vi "二进制文件读取.vi"() -> ()   [LabVIEW 2018]
panel:
  out "数据 2":i32[](array[numeric])
  in  "path":path caption="路径"
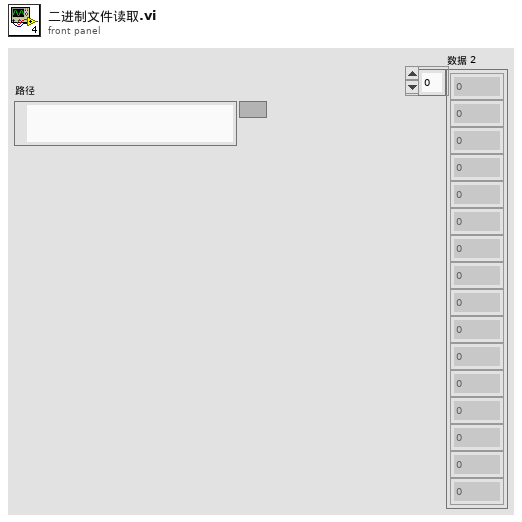
[diagram p1: front panel]
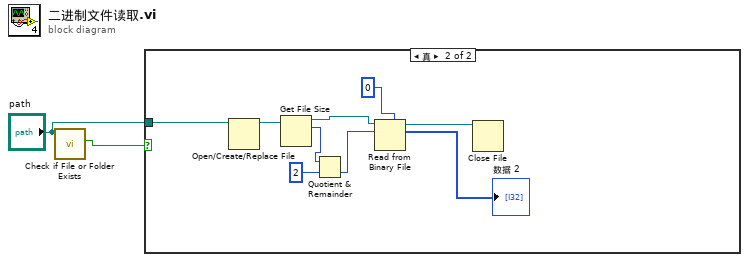
[diagram p0: block diagram]
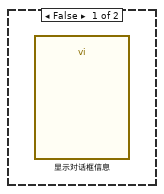
[diagram p2: hidden frame]
diagram:
  n1 = call <vilib>:"Check if File or Folder Exists.vi"("path"="path") -> ("file or folder exists?"=w2:bool)  [unwired: 8 in, 2 out]
  n2 = case shown="真" w2 {
    tunnel: "path" -> [_ w11]
    frame False {
      n3 = call "显示对话框信息"() -> ()  [unwired: 10 in, 2 out]
    }
    frame True {
      n4 = Open/Create/Replace File(file path (use dialog)=w11) -> (refnum out=w8:refnum<file>)  [unwired: 5 in, 2 out]
      n5 = Get File Size(file=w8) -> (refnum out=w7:refnum<file>, size (in bytes)=w6:i64)  [unwired: 1 in, 1 out]
      n6 = Quotient & Remainder(x=w6, y=i64 2) -> (floor(x/y)=w4:i64)  [unwired: 1 out]
      n7 = Read from Binary File(5:i16 0, 10:w4, 11:w7) -> (2:→"数据 2":i16[], 3:w10:refnum<file>)  [unwired: 3 in, 2 out]
      n8 = Close File(refnum=w10) -> ()  [unwired: 1 in, 2 out]
    }
  }
